vi "SetControlsFromVariant.vi"(8 "error in":errorcluster, 10 "Variant Array":variant[](array[variant]), 11 "Controls[] in":refnum<vi>[](array[refnum])) -> (0 "error out":errorcluster, 3 "Controls[] out":refnum<vi>[](array[refnum]))   [LabVIEW 2012]
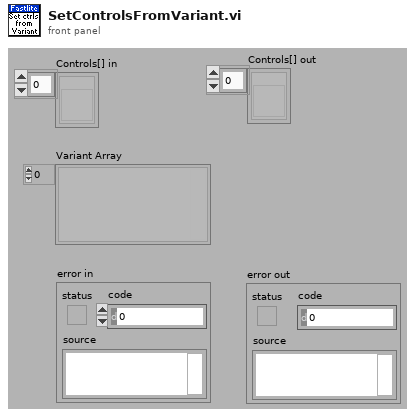
[diagram p1: front panel]
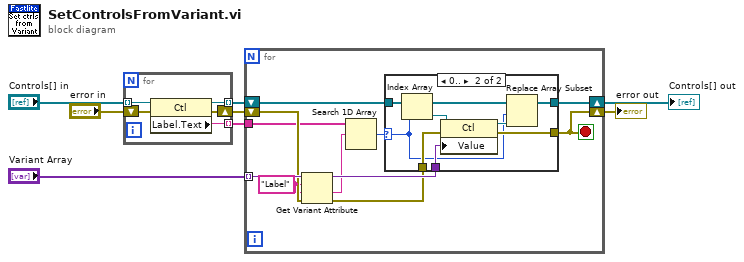
[diagram p0: block diagram]
diagram:
  n1 = for {
    tunnel: "Controls[] in" -> [w13] mode=indexing
    tunnel: [w12] -> w7 mode=indexing
    tunnel: [w11] -> w8 mode=indexing
    shift-right: [w9] -> w5
    shift-left: "error in" -> [w10]
    n2 = property class="Ctl"(reference=w13, error in=w10) -> (reference out=w11:refnum<vi>, error out=w9:errorcluster, "Label.Text"=w12:string)
  }
  n3 = for {
    tunnel: w7 -> [w21]
    tunnel: "Variant Array" -> [w24] mode=indexing
    shift-right: [w16] -> w2
    shift-left: w5 -> [w23]
    shift-right: [w17] -> w1
    shift-left: w8 -> [w20]
    stop <- w16 stop-if-true
    w22 = "Label" ("name")
    n4 = Get Variant Attribute(Variant=w24, name=w22, default value (empty Variant)=w22, error in=w23) -> (duplicate Variant=w19:variant, value=w15:string, error out=w18:errorcluster)  [unwired: 1 out]
    n5 = Search 1D Array(1D array=w21, element=w15) -> (index of element=w14:i32)  [unwired: 1 in]
    n6 = case shown="0.." w14 {
      selector: w14 -> [_ w27]
      tunnel: w20 -> [w25 w33]
      tunnel: w19 -> [_ w31]
      tunnel: w18 -> [w26 w30]
      tunnel: [w25 w29] -> w17
      tunnel: [w26 w28] -> w16
      frame ..-1 {
      }
      frame 0.. {
        n7 = Index Array(array=w33, index=w27) -> (element=w34:refnum<vi>)
        n8 = property class="Ctl"(reference=w34, error in=w30, "Value"=w31) -> (reference out=w32:refnum<vi>, error out=w28:errorcluster)
        n9 = Replace Array Subset(array=w33, new element=w32, index=w27) -> (w29:refnum<vi>[])
      }
    }
  }
  "error out" <- w2
  "Controls[] out" <- w1
